vi "Sample Rate To Loop Time (us).vi"(0 "sample rate (S/s)":dbl format="%#_6p", 1 "FPGA clock rate (Hz)":dbl=40000000.0 format="%#_6p", 11 "error in (no error)":errorcluster) -> (4 "count (us/S)":u32, 10 "actual sample rate (S/s)":dbl format="%#_6p", 15 "error out":errorcluster)   [LabVIEW 2020, in "NI_FpgaMspHost.lvlib"]
doc: "Converts the desired sample rate to the appropriate count for the Loop Timer Express VI and computes the achievable sample rate for use with other Scaling VIs."
uses:
  <vilib>/rvi/Analysis/host/Public/NI_FpgaMspHost.lvlib
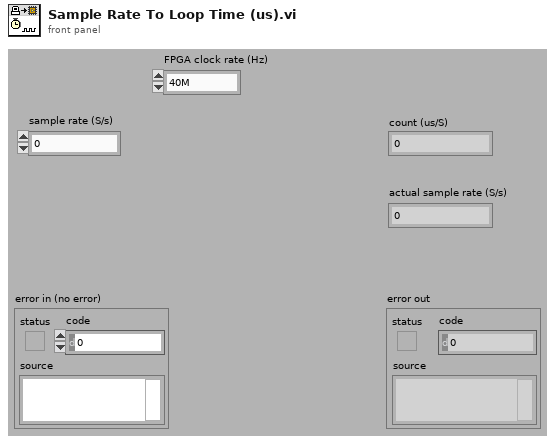
[diagram p1: front panel]
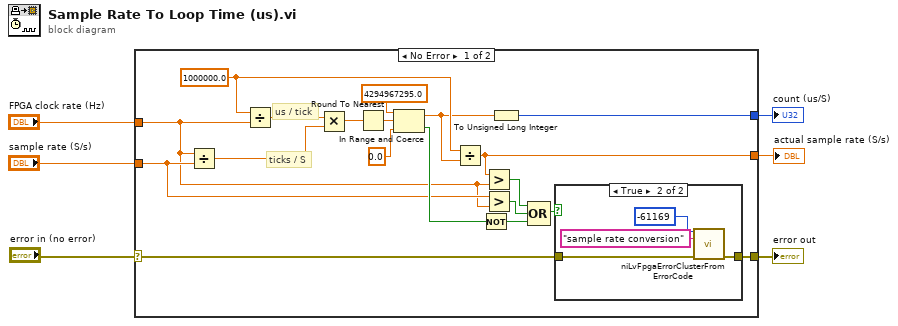
[diagram p0: block diagram]
diagram:
  n1 = case shown="No Error" "error in (no error)" {
    selector: "error in (no error)" -> [w22 w31]
    tunnel: "FPGA clock rate (Hz)" -> [w10 _]
    tunnel: "sample rate (S/s)" -> [w11 _]
    tunnel: [w21 _] -> w3
    tunnel: [w15 _] -> w1
    tunnel: [w23 w31] -> w2
    frame No Error {
      w20 = 1000000.0 ("x")
      # "ticks / S"
      # "us / tick"
      n2 = Divide(x=w10, y=w11) -> (x/y=w24:dbl)
      n3 = Divide(x=w20, y=w10) -> (x/y=w25:dbl)
      n4 = Multiply(x=w25, y=w24) -> (x*y=w8:dbl)
      n5 = Round To Nearest(number=w8) -> (nearest integer value=w7:dbl)
      n6 = In Range and Coerce(upper limit=4294967295.0 ("unsigned 32bit integer"), x=w7, lower limit=0.0) -> (coerced(x)=w9:dbl, In Range?=w17:bool)
      n7 = Divide(x=w20, y=w9) -> (x/y=w15:dbl)
      n8 = Not(x=w17) -> (.not. x?=w13:bool)
      n9 = Greater?(x=w15, y=w10) -> (0:w14:bool)
      n10 = Greater?(x=w11, y=w10) -> (0:w12:bool)
      n11 = To Unsigned Long Integer(number=w9) -> (unsigned 32bit integer=w21:u32)
      n12 = Compound Arithmetic op=OR(w14, w12, w13) -> (w16:bool)
      n13 = case shown="True" w16 {
        tunnel: [w26 w30] -> w23
        tunnel: w22 -> [w26 w27]
        frame False {
        }
        frame True {
          n14 = call <vilib>:"niLvFpgaErrorClusterFromErrorCode.vi"("error code"=-61169, "function name"="sample rate conversion" ("L10N_Function Name"), "error in"=w27) -> ("error out"=w30:errorcluster)  [unwired: 4 in, 8 out]
        }
      }
    }
    frame Error {
    }
  }
  "error out" <- w2
  "count (us/S)" <- w3
  "actual sample rate (S/s)" <- w1
